vi "test.vi"() -> ()   [LabVIEW 2010]
uses:
  MagiQmw3.lvclass
panel:
  out "Updates":i32
  in  "Enable":bool=TRUE
  in  "Ch":i32=2 min=0 max=2
  in  "Atten (dB)":dbl
  in  "Frequency (MHz)":dbl=100.0
  in  "stop":bool
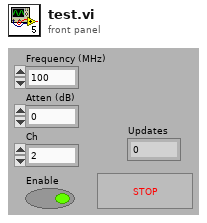
[diagram p1: front panel]
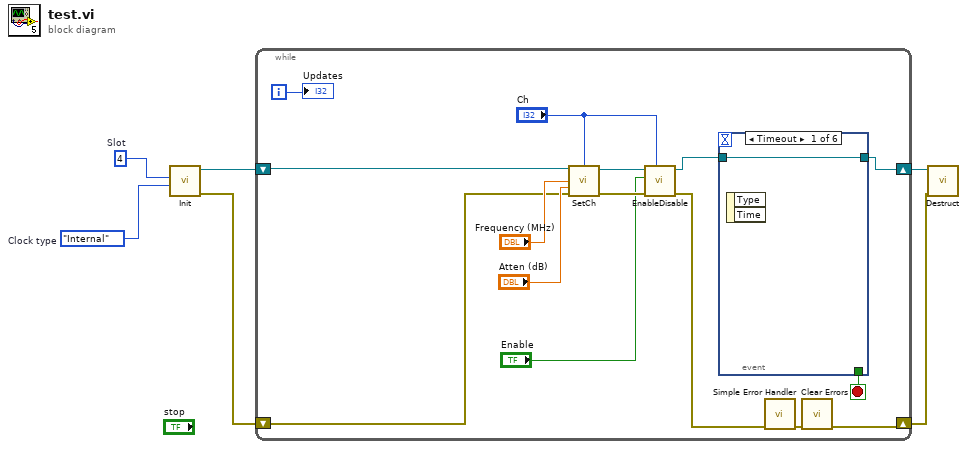
[diagram p0: block diagram]
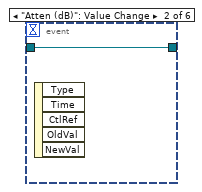
[diagram p2: hidden frame]
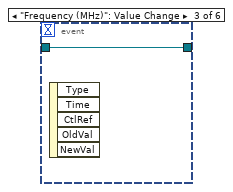
[diagram p3: hidden frame]
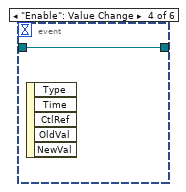
[diagram p4: hidden frame]
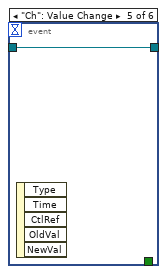
[diagram p5: hidden frame]
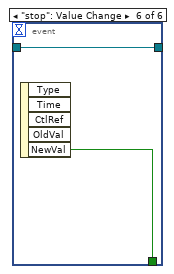
[diagram p6: hidden frame]
diagram:
  w5 = u16 4  # Slot
  w6 = enum8{"Internal", "External", "PXI"}."Internal"  # Clock type
  n1 = call "Init.vi"("Clock type"=w6, "Slot"=w5) -> ("error out"=w2:errorcluster, "MagiQmw3 out"=w1:refnum<class "MagiQmw3.lvclass">)  [unwired: 8 in]
  n2 = while {
    shift-right: [w7] -> w3
    shift-left: w2 -> [w14]
    shift-right: [w11] -> w4
    shift-left: w1 -> [w10]
    i -> [w15]
    stop <- w13 stop-if-true
    n3 = call "SetCh.vi"("MagiQmw3 in"=w10, "ch"="Ch", "freq"="Frequency (MHz)", "atten"="Atten (dB)", "error in (no error)"=w14) -> ("MagiQmw3 out"=w19:refnum<class "MagiQmw3.lvclass">, "error out"=w18:errorcluster)  [unwired: 9 in]
    n4 = call "EnableDisable.vi"("ch"="Ch", "error in (no error)"=w18, "Enable"="Enable", "MagiQmw3 in"=w19) -> ("error out"=w9:errorcluster, "MagiQmw3 out"=w12:refnum<class "MagiQmw3.lvclass">)  [unwired: 6 in]
    n5 = event shown="[0] Timeout" {
      selector: _ -> [_ _ _ _ _ _]
      dyn-events: _ -> [_ _ _ _ _ _]
      timeout: _ -> [_ _ _ _ _ _]
      tunnel: w12 -> [w22 w23 w24 w25 w26 w28]
      tunnel: [w22 w23 w24 w25 w26 w28] -> w11
      tunnel: [_ _ _ _ _ w27] -> w13
      event Timeout {
        n6 = event-data() -> ()  [unwired: 1 in, 2 out]
      }
      event "Atten (dB)": Value Change {
        n7 = event-data() -> ()  [unwired: 1 in, 5 out]
      }
      event "Frequency (MHz)": Value Change {
        n8 = event-data() -> ()  [unwired: 1 in, 5 out]
      }
      event "Enable": Value Change {
        n9 = event-data() -> ()  [unwired: 1 in, 5 out]
      }
      event "Ch": Value Change {
        n10 = event-data() -> ()  [unwired: 1 in, 5 out]
      }
      event "stop": Value Change {
        n11 = event-data() -> ("NewVal"=w27:bool)  [unwired: 1 in, 4 out]
      }
    }
    n12 = call <vilib>:"Simple Error Handler.vi"("error in (no error)"=w9) -> ("error out"=w8:errorcluster)  [unwired: 4 in, 4 out]
    n13 = call <vilib>:"Clear Errors.vi"("error in (no error)"=w8) -> ("error out"=w7:errorcluster)  [unwired: 6 in]
    "Updates" <- w15
  }
  n14 = call "Destruct.vi"("error in (no error)"=w3, "MagiQmw3 in"=w4) -> ()  [unwired: 9 in, 1 out]
